vi "ke37xx Scan List Example.vi"() -> ()   [LabVIEW 2009]
doc: "Scan List Example\n \nThis sample demonstrates use of the Ke37XX scanning features.\nA set of channels is used to configure the scan list and then\na measurement function is specified. \nThe measurement function is performed for each channel in the\nscan list and the results are presented in a string indicator\non the front panel. Note that the \"# Channels\" control must \nmatch the actual number of channels represented in the channel\nlist specified. Finally, the scan count can be used to control\nhow many times the Ke37XX iterates through the scan list.\n\nUse of Pseudo Cards\n\nThis sample can be run using a mainframe that has no cards\npresent in the system slots (1 to 6). This is accomplished\nby use of the Ke37XX's native support for \"pseudo cards\".\nBy using pseudo cards, instrument commands may be sent to\nthe Ke37XX as if the cards were physically present. The \ninstrument responses will be simulated by the instrument itself.\nCombo boxes are provided for specifying which card should be\nsimulated in each slot."
uses:
  <instrlib>/Keithley 3706/Keithley 3700 Series.lvlib
panel:
  out "Readings":dbl[](array[numeric]) format="%#_6e"
  in  "Scan Count":u32=3
  in  "# Channels":u32=5
  in  "Scan List":string="1001:1005"
  in  "Measurement Function":string="dcvolts"
  in  "Slot 6 Pseudocard (6: 3740)":u16(ring)=5 items=["Empty", "3720", "3721", "3722", "3723", "3730", "3740"]
  in  "Slot 5 Pseudocard (5: 3730)":u16(ring)=5 items=["Empty", "3720", "3721", "3722", "3723", "3730", "3740"]
  in  "Slot 4 Pseudocard (4: 3723)":u16(ring)=4 items=["Empty", "3720", "3721", "3722", "3723", "3730", "3740"]
  in  "Slot 3 Pseudocard (3: 3722)":u16(ring)=3 items=["Empty", "3720", "3721", "3722", "3723", "3730", "3740"]
  in  "Slot 2 Pseudocard (2: 3721)":u16(ring)=2 items=["Empty", "3720", "3721", "3722", "3723", "3730", "3740"]
  in  "Slot 1 Pseudocard (1: 3720)":u16(ring)=1 items=["Empty", "3720", "3721", "3722", "3723", "3730", "3740"]
  in  "VISA Resource Name":refnum<visa-resource-name>="GPIB::6"
  # "Each measurement will be taken for each channel in the scan list."
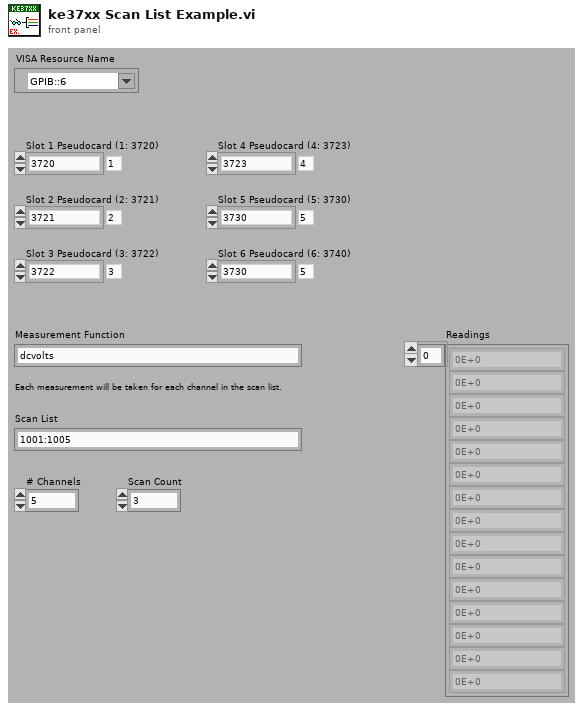
[diagram p1: front panel]
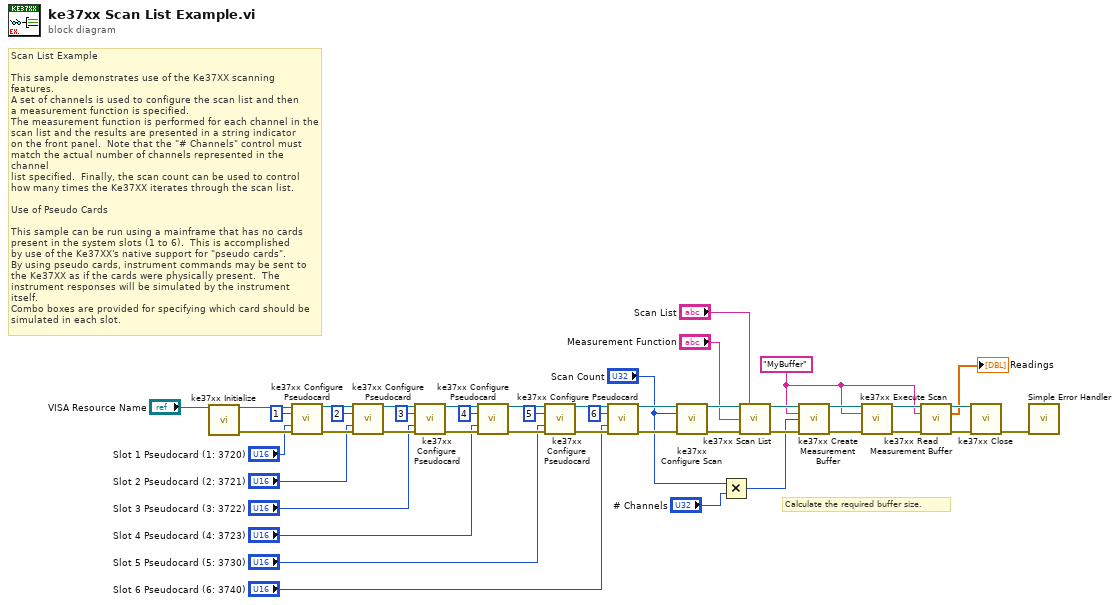
[diagram p0: block diagram]
diagram:
  w10 = "MyBuffer" ("Buffer Name")
  # "Calculate the required buffer size."
  # "Scan List Example\n \nThis sample demonstrates use of the Ke37XX scanning features.\nA set of channels is used to configure the scan list and then\na measurement function is specified.  \nThe measurement function is performed for each channel in the\nscan list and the results are presented in a string indicator\non the front panel.  Note that the \"# Channels\" control must \nmatch the actual number of channels represented in the channel\nlist specified.  Finally, the scan count can be used to control\nhow many times the Ke37XX iterates through the scan list.\n\nUse of Pseudo Cards\n\nThis sample can be run using a mainframe that has no cards\npresent in the system slots (1 to 6).  This is accomplished\nby use of the Ke37XX's native support for \"pseudo cards\".\nBy using pseudo cards, instrument commands may be sent to\nthe Ke37XX as if the cards were physically present.  The \ninstrument responses will be simulated by the instrument itself.\nCombo boxes are provided for specifying which card should be\nsimulated in each slot."
  n1 = call <instrlib>:"ke37xx Initialize.vi"("VISA resource name"="VISA Resource Name") -> ("VISA resource name out"=w18:refnum<visa-resource-name>, "error out"=w43:errorcluster)  [unwired: 13 in]
  n2 = call <instrlib>:"ke37xx Configure Pseudocard.vi"("VISA Resource Name"=w18, "Slot Number (1)"=1, "Pseudocard Name (1: 3720)"="Slot 1 Pseudocard (1: 3720)", "error in (no error)"=w43) -> ("VISA Resource Name Out"=w34:refnum<visa-resource-name>, "error out"=w28:errorcluster)  [unwired: 10 in]
  n3 = call <instrlib>:"ke37xx Configure Pseudocard.vi"("VISA Resource Name"=w34, "Slot Number (1)"=2, "Pseudocard Name (1: 3720)"="Slot 2 Pseudocard (2: 3721)", "error in (no error)"=w28) -> ("VISA Resource Name Out"=w33:refnum<visa-resource-name>, "error out"=w27:errorcluster)  [unwired: 10 in]
  n4 = call <instrlib>:"ke37xx Configure Pseudocard.vi"("VISA Resource Name"=w33, "Slot Number (1)"=3, "Pseudocard Name (1: 3720)"="Slot 3 Pseudocard (3: 3722)", "error in (no error)"=w27) -> ("VISA Resource Name Out"=w32:refnum<visa-resource-name>, "error out"=w26:errorcluster)  [unwired: 10 in]
  n5 = call <instrlib>:"ke37xx Configure Pseudocard.vi"("VISA Resource Name"=w32, "Slot Number (1)"=4, "Pseudocard Name (1: 3720)"="Slot 4 Pseudocard (4: 3723)", "error in (no error)"=w26) -> ("VISA Resource Name Out"=w31:refnum<visa-resource-name>, "error out"=w25:errorcluster)  [unwired: 10 in]
  n6 = call <instrlib>:"ke37xx Configure Pseudocard.vi"("VISA Resource Name"=w31, "Slot Number (1)"=5, "Pseudocard Name (1: 3720)"="Slot 5 Pseudocard (5: 3730)", "error in (no error)"=w25) -> ("VISA Resource Name Out"=w30:refnum<visa-resource-name>, "error out"=w24:errorcluster)  [unwired: 10 in]
  n7 = call <instrlib>:"ke37xx Configure Pseudocard.vi"("VISA Resource Name"=w30, "Slot Number (1)"=6, "Pseudocard Name (1: 3720)"="Slot 6 Pseudocard (6: 3740)", "error in (no error)"=w24) -> ("VISA Resource Name Out"=w17:refnum<visa-resource-name>, "error out"=w16:errorcluster)  [unwired: 10 in]
  n8 = call <instrlib>:"ke37xx Configure Scan.vi"("VISA Resource Name"=w17, "Scan Count (1)"="Scan Count", "error in (no error)"=w16) -> ("VISA Resource Name Out"=w15:refnum<visa-resource-name>, "error out"=w14:errorcluster)  [unwired: 11 in]
  n9 = Multiply(x="Scan Count", y="# Channels") -> (x*y=w3:u32)
  n10 = call <instrlib>:"ke37xx Scan List.vi"("VISA Resource Name"=w15, "Channel List"="Scan List", "Configuration"="Measurement Function", "error in (no error)"=w14) -> ("VISA Resource Name Out"=w45:refnum<visa-resource-name>, "error out"=w9:errorcluster)  [unwired: 9 in, 1 out]
  n11 = call <instrlib>:"ke37xx Create Measurement Buffer.vi"("VISA Resource Name"=w45, "Buffer Name"=w10, "Capacity"=w3, "error in (no error)"=w9) -> ("VISA Resource Name Out"=w12:refnum<visa-resource-name>, "error out"=w8:errorcluster)  [unwired: 10 in]
  n12 = call <instrlib>:"ke37xx Execute Scan.vi"("VISA Resource Name"=w12, "Buffer Name"=w10, "error in (no error)"=w8) -> ("VISA Resource Name Out"=w11:refnum<visa-resource-name>, "error out"=w7:errorcluster)  [unwired: 11 in]
  n13 = call <instrlib>:"ke37xx Read Measurement Buffer.vi"("VISA Resource Name"=w11, "Buffer Name"=w10, "error in (no error)"=w7) -> ("VISA Resource Name Out"=w44:refnum<visa-resource-name>, "Readings"=→"Readings":dbl[], "error out"=w2:errorcluster)  [unwired: 6 in, 4 out]
  n14 = call <instrlib>:"ke37xx Close.vi"("VISA resource name"=w44, "error in (no error)"=w2) -> ("error out"=w41:errorcluster)  [unwired: 13 in]
  n15 = call <vilib>:"Simple Error Handler.vi"("error in (no error)"=w41) -> ()  [unwired: 1 in, 8 out]
